vi "Get_PN.vi"(8 "error in (no error)":errorcluster caption="entrée d'erreur (pas d'erreur)", 11 "Class Creation_SN (Default) en entrée":refnum<class "Creation_SN Database (Default).lvclass">) -> (0 "error out":errorcluster caption="sortie d'erreur", 3 "Class Creation_SN (Default) en sortie":refnum<class "Creation_SN Database (Default).lvclass">)   [LabVIEW 2020, in "Library Instrument & Equipement.lvlib" / "Library Creation_SN.lvlib" / "Creation_SN Database (Default).lvclass"]
uses:
  Creation_SN Database (Default).lvclass
  Instrument/Instrument Firebase Altyor/Class Instrument Firebase Altyor.lvclass
  Creation_SN Database (Default).lvclass/Creation_SN Database (Default).ctl
  Commun VI/TypeDef/Variable Printable.ctl
  Firebase/Source/Firebase Recovery_SN/Firebase Recovery_SN.lvclass
  C:/Users/ngarcin/OneDrive - Altyor/Standard TB/Suite TB45/Class/Firebase/Source/Firebase Driver/Firebase Driver.lvclass
  Commun VI/Library Commun.lvlib
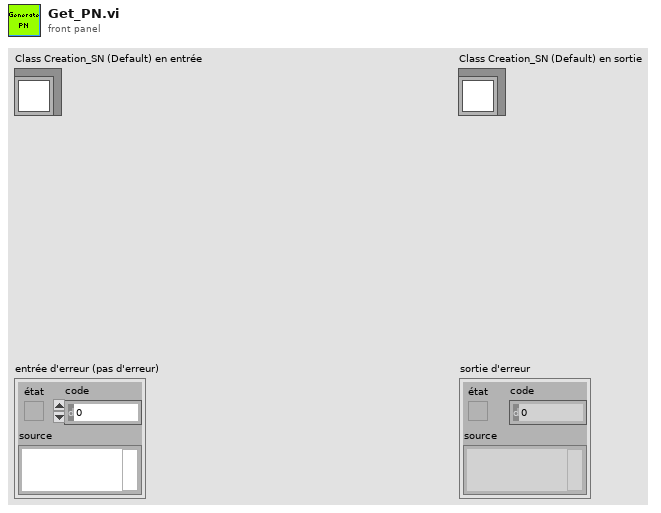
[diagram p1: front panel]
types:
  T1 = enum16{"Get Variable", "Get All Variables", "Set Variable", "Delete Variable", "Delete All Variable"}
  T2 = typedef "Variable Printable.ctl" = string
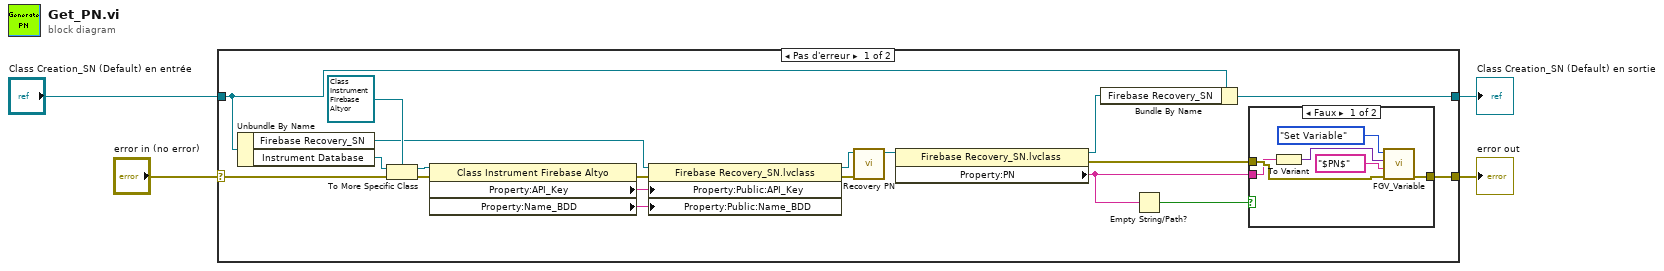
[diagram p0: block diagram]
diagram:
  n1 = case shown="Pas d'erreur" "error in (no error)" {
    selector: "error in (no error)" -> [w15 w32]
    tunnel: [w11 w32] -> w3
    tunnel: [w14 w31] -> w1
    tunnel: "Class Creation_SN (Default) en entrée" -> [w23 w31]
    frame No Error {
      n2 = Unbundle By Name(w23) -> ("Firebase Recovery_SN"=w7:refnum<class "Firebase Recovery_SN.lvclass">, "Instrument Database"=w16:refnum<class "Class Instrument (Default).lvclass">)
      n3 = To More Specific Class(target class=refnum<class "Class Instrument Firebase Altyor.lvclass"> refnum ("Library Instruments.lvlib:Class Instrument Firebase Altyor.lvclass"), reference=w16, error in=w15) -> (specific class reference=w20:refnum<class "Class Instrument Firebase Altyor.lvclass">, error out=w21:errorcluster)
      n4 = property class="Class Instrument Firebase Altyo"(reference=w20, error in=w21) -> (error out=w19:errorcluster, "Property:API_Key"=w18:string, "Property:Name_BDD"=w17:string)  [unwired: 1 out]
      n5 = property class="Firebase Recovery_SN.lvclass"(reference=w7, error in=w19, "Property:Public:API_Key"=w18, "Property:Public:Name_BDD"=w17) -> (reference out=w12:refnum<class "Firebase Recovery_SN.lvclass">, error out=w13:errorcluster)
      n6 = call-dynamic "Recovery PN.vi"("error in (no error)"=w13, "Firebase Benches en entrée"=w12) -> ("Firebase Benches en sortie"=w10:refnum<class "Firebase Recovery_SN.lvclass">)  [unwired: 8 in, 1 out]
      n7 = property class="Firebase Recovery_SN.lvclass"(reference=w10) -> (reference out=w9:refnum<class "Firebase Recovery_SN.lvclass">, error out=w8:errorcluster, "Property:PN"=w6:string)  [unwired: 1 in]
      n8 = Bundle By Name(cluster=w23, "Firebase Recovery_SN"=w9) -> (w14:refnum<class "Creation_SN Database (Default).lvclass">)
      n9 = Empty String/Path?(string/path=w6) -> (empty?=w5:bool)
      n10 = case shown="Faux" w5 {
        tunnel: [w26 w30] -> w11
        tunnel: w8 -> [w25 w30]
        tunnel: w6 -> [w24 _]
        frame False {
          n11 = To Variant(anything=w24) -> (Variant=w27:variant)
          n12 = call "FGV_Variable.vi"("error in (no error)"=w25, "Variable"=T2 "$PN$" ("Variable Printable"), "Data In"=w27, "Function"=T1."Set Variable") -> ("error out"=w26:errorcluster)  [unwired: 5 in, 2 out]
        }
        frame True {
        }
      }
    }
    frame Error {
    }
  }
  "error out" <- w3
  "Class Creation_SN (Default) en sortie" <- w1
